vi "Is PM Active.vi"(8 "error in (no error)":errorcluster) -> (0 "error out":errorcluster, 3 "FAC PM User Event":refnum<user-event>)   [LabVIEW 2018, in "Assert API Components.lvlib" / "Process Monitor.lvlib"]
uses:
  Process Monitor.lvlib
  PM_Data.ctl
  Core/Assert API Components/Log Assert Core Components/Event Transmission/Failure Action Change Event Reference.ctl
  Core/Assert API Components/Log Assert Core Components/Log Assert Core.lvlib
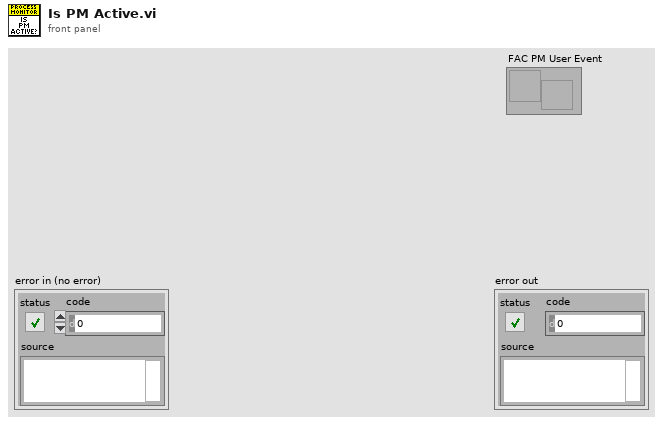
[diagram p1: front panel]
types:
  T1 = enum32{"Bad", "Idle", "Run top level", "Running"}
  T2 = typedef "Assert API Components.lvlib/Process Monitor.lvlib/PM_Data.ctl" = cluster{"Caller VI Name":string, "Failure Action Event References":T3, "MD5":string}
  T3 = typedef "Assert API Components.lvlib/Log Assert Core.lvlib/Failure Action Change Event Reference.ctl" = cluster{"Failure Action Change Event":refnum<user-event>, "Event Registration Refnum":refnum<event-registration>}
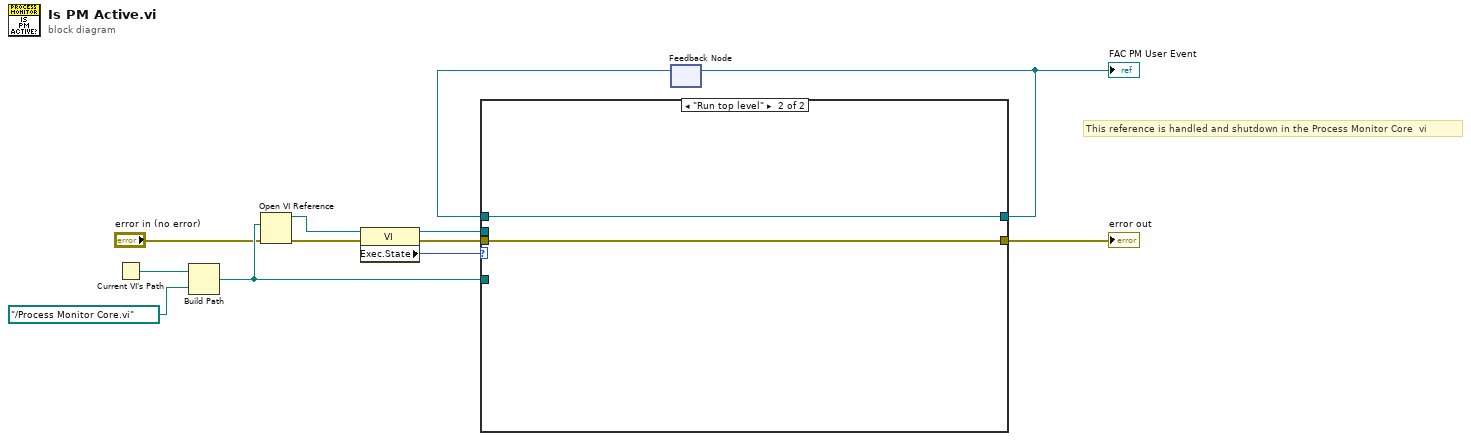
[diagram p0: block diagram]
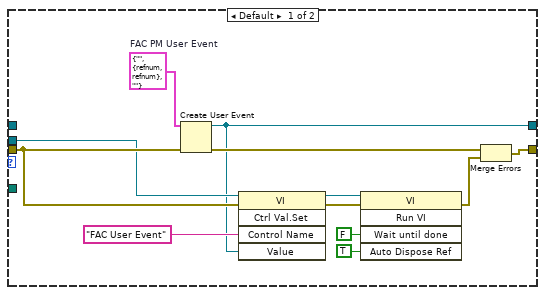
[diagram p2: hidden frame]
diagram:
  # "This reference is handled and shutdown in the Process Monitor Core  vi"
  n1 = Current VI's Path() -> (path=w4:path)
  n2 = Build Path(base path=w4, name or relative path=path "../Process Monitor Core.vi" ("VI Path")) -> (appended path=w3:path)
  n3 = Open VI Reference(vi path=w3, error in (no error)="error in (no error)") -> (vi reference=w11:refnum<vi>, error out=w12:errorcluster)  [unwired: 4 in]
  n4 = property class="VI"(reference=w11, error in=w12) -> (reference out=w1:refnum<vi>, error out=w9:errorcluster, "Exec.State"=w10:T1)
  n5 = feedback #1() -> (w7:refnum<user-event>)  [unwired: 1 in]
  n6 = case shown="\"Run top level\"" w10 {
    tunnel: w9 -> [w21 w25]
    tunnel: [w13 w26] -> w8
    tunnel: w7 -> [_ w26]
    tunnel: [w22 w25] -> w6
    tunnel: w3 -> [_ _]
    tunnel: w1 -> [w17 _]
    frame Default {
      w24 = T2 {"Caller VI Name"="", "Failure Action Event References"={"Failure Action Change Event"=refnum, "Event Registration Refnum"=refnum}, "MD5"=""}  # FAC PM User Event
      n7 = Create User Event(user event datatype=w24, error in=w21) -> (user event=w13:refnum<user-event>, error out=w20:errorcluster)
      n8 = invoke class="VI" method="Ctrl Val.Set"(reference=w17, error in=w21, "Control Name"="FAC User Event", "Value"=w13) -> (reference out=w18:refnum<vi>, error out=w23:errorcluster)  [unwired: 1 in, 3 out]
      n9 = invoke class="VI" method="Run VI"(reference=w18, error in=w23, "Wait until done"=FALSE ("Wait Until Done"), "Auto Dispose Ref"=TRUE ("Auto Dispose Reference")) -> (error out=w19:errorcluster)  [unwired: 1 in, 4 out]
      n10 = Merge Errors(w20, w19) -> (w22:errorcluster)
    }
    frame "Run top level" {
    }
  }
  "error out" <- w6
  "FAC PM User Event" <- w8
  n11 = feedback-in #1(w8) -> ()
